vi "Email_With_Log.vi"(0 "recipients":string[](array[string]), 1 "subject ([No Subject])":string="[No Subject]", 2 "message":string, 3 "attachments":T1(array[cluster])) -> (5 "invalid recipients":string[](array[string]), 6 "error out":errorcluster)   [LabVIEW 2010]
uses:
  Globals/Preference_global.vi
  Globals/Constants_global.vi
  <vilib>/Utility/SMTP/NI_SMTPEmail.lvlib
panel:
  out "Number of valid email requests":i32
  # "Image/x-png"
  # "Image/jpeg"
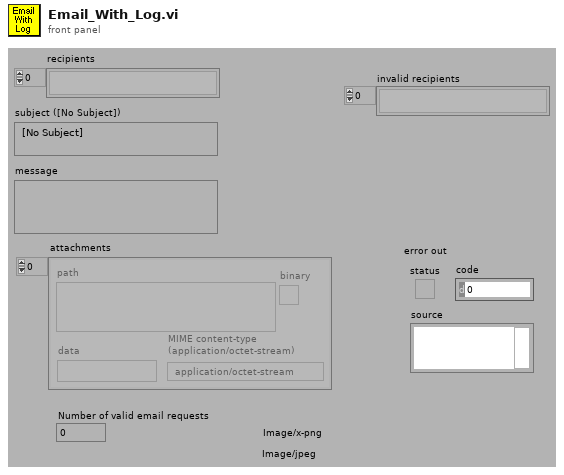
[diagram p1: front panel]
types:
  T1 = cluster{"path":path, "data":string, "binary":bool, "MIME content-type \n(application/octet-stream)":string}[]
  T2 = cluster{"path":path, "data":string, "binary":bool, "MIME content-type \n(application/octet-stream)":string}
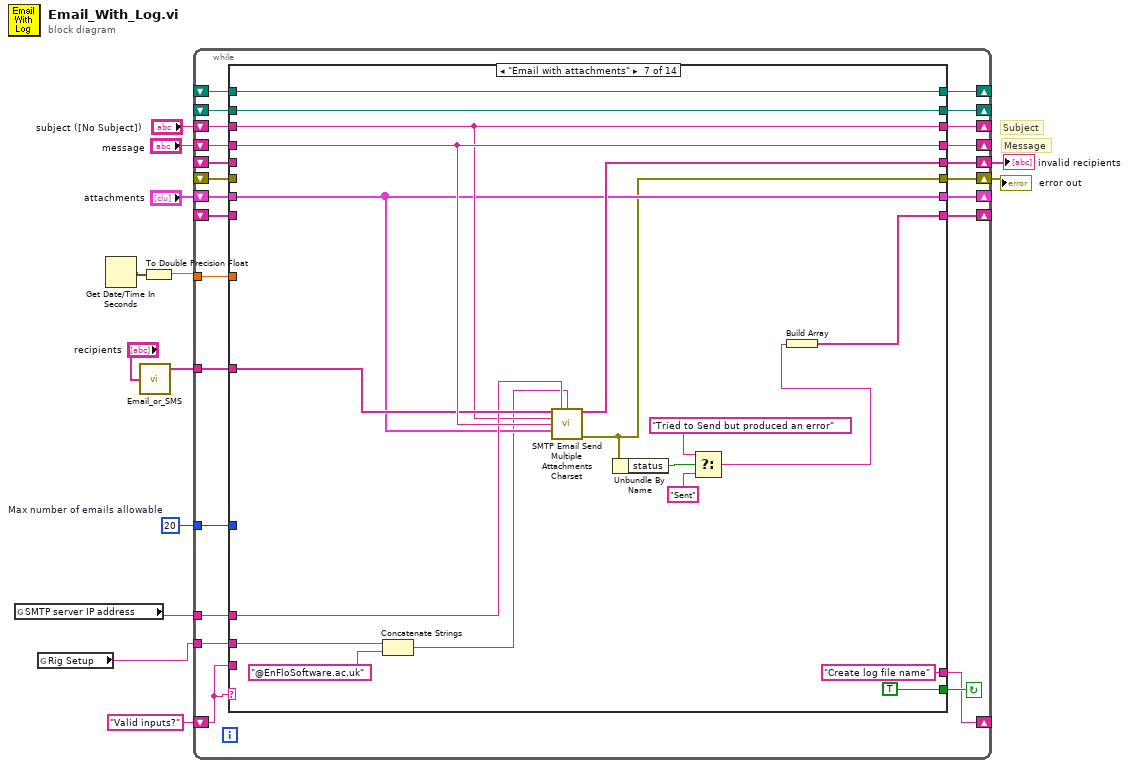
[diagram p0: block diagram]
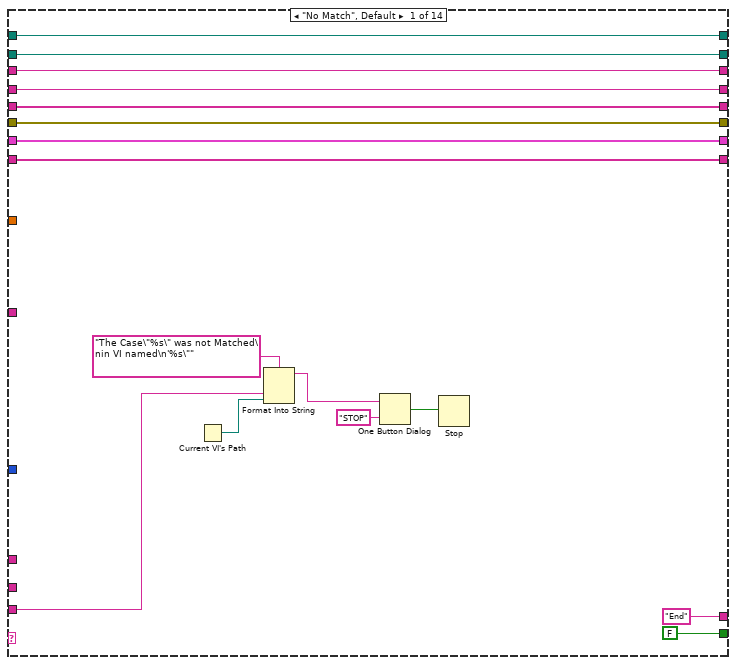
[diagram p2: hidden frame]
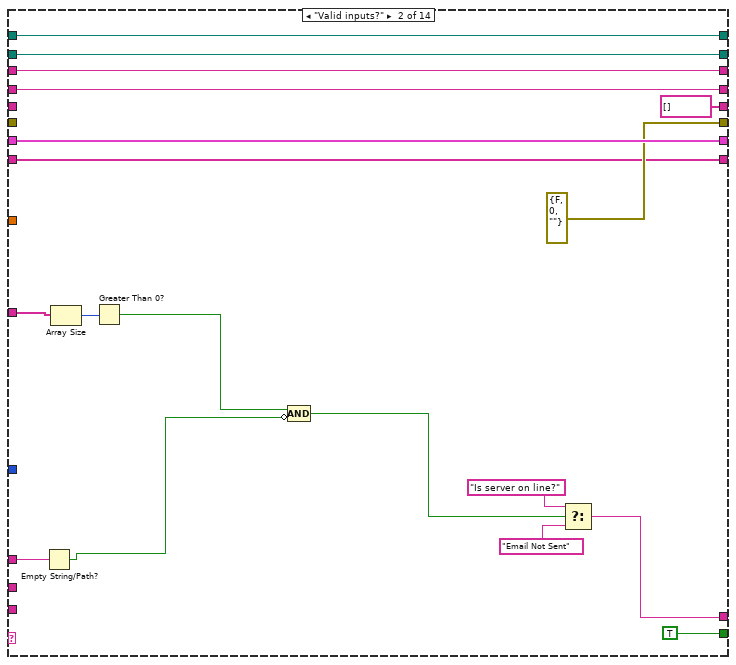
[diagram p3: hidden frame]
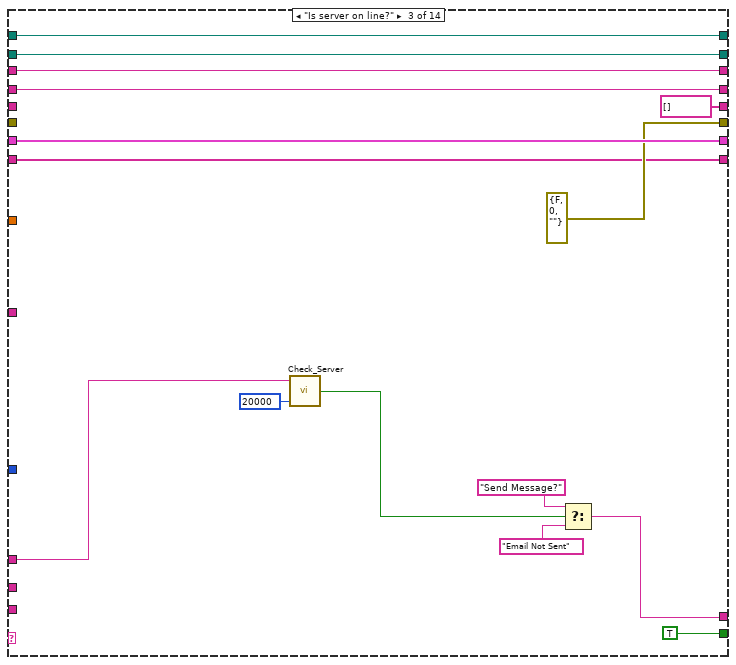
[diagram p4: hidden frame]
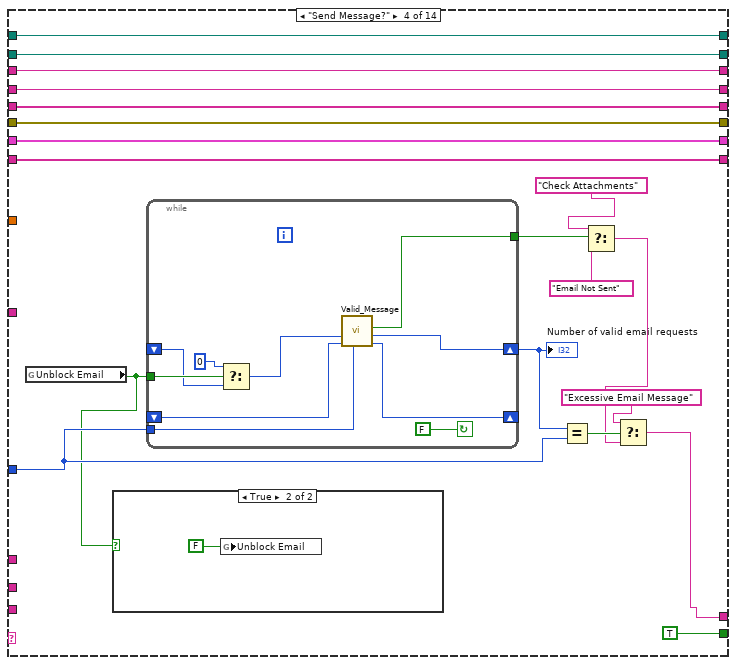
[diagram p5: hidden frame]
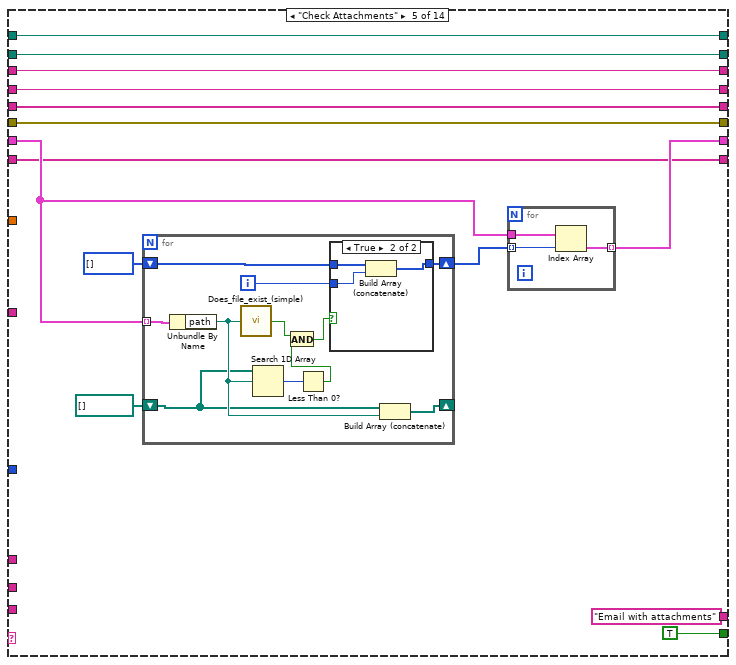
[diagram p7: hidden frame]
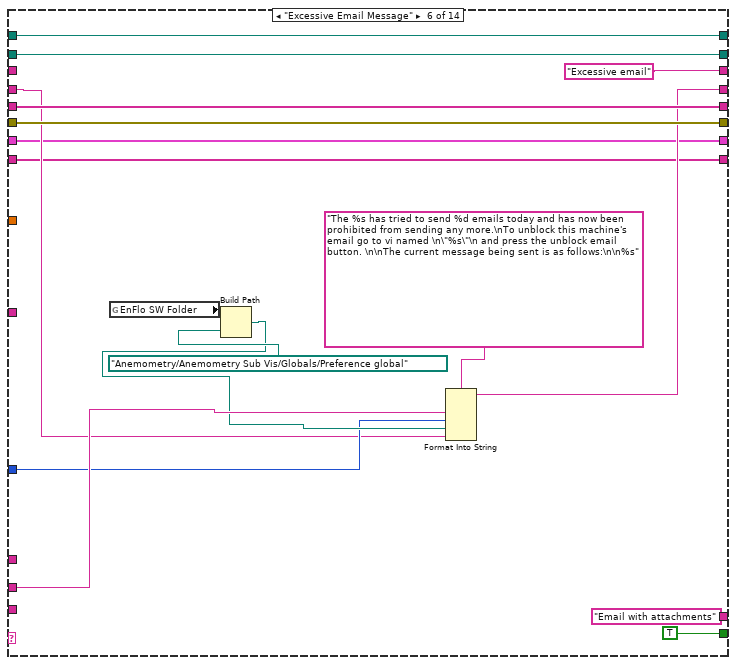
[diagram p9: hidden frame]
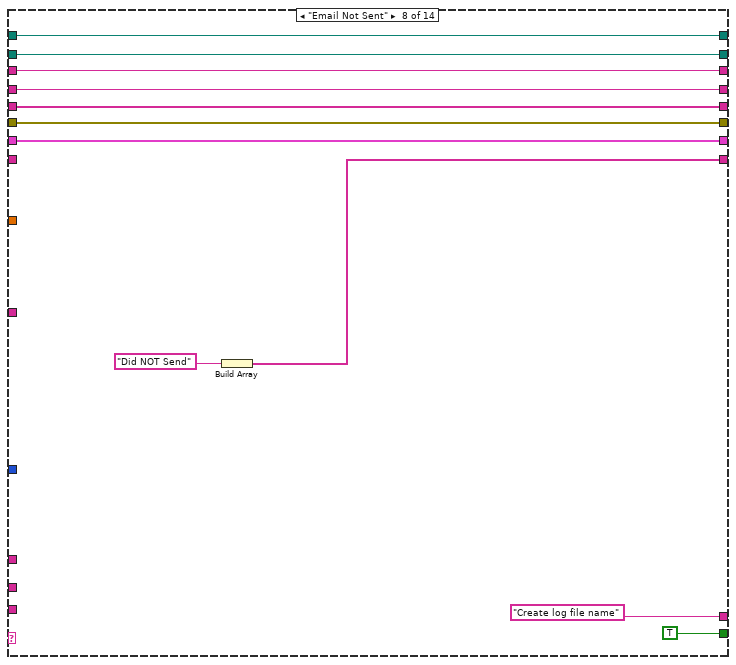
[diagram p10: hidden frame]
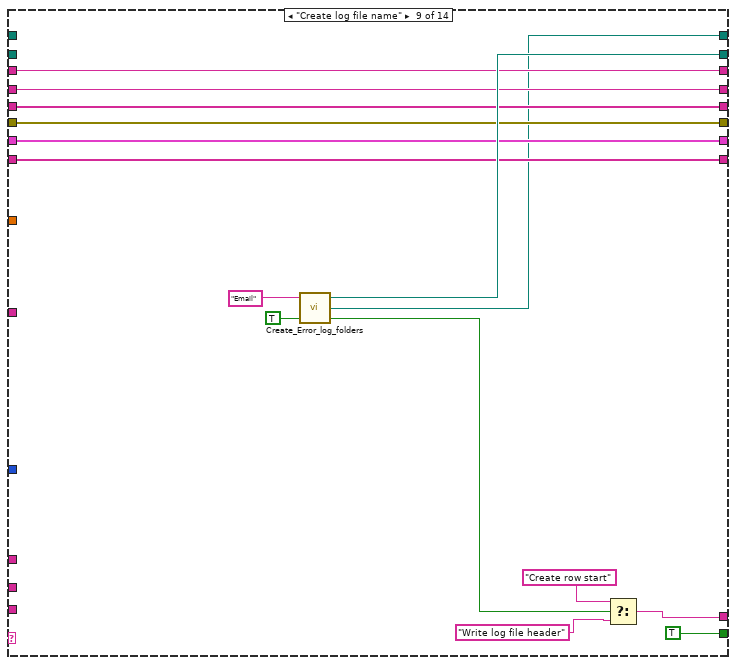
[diagram p11: hidden frame]
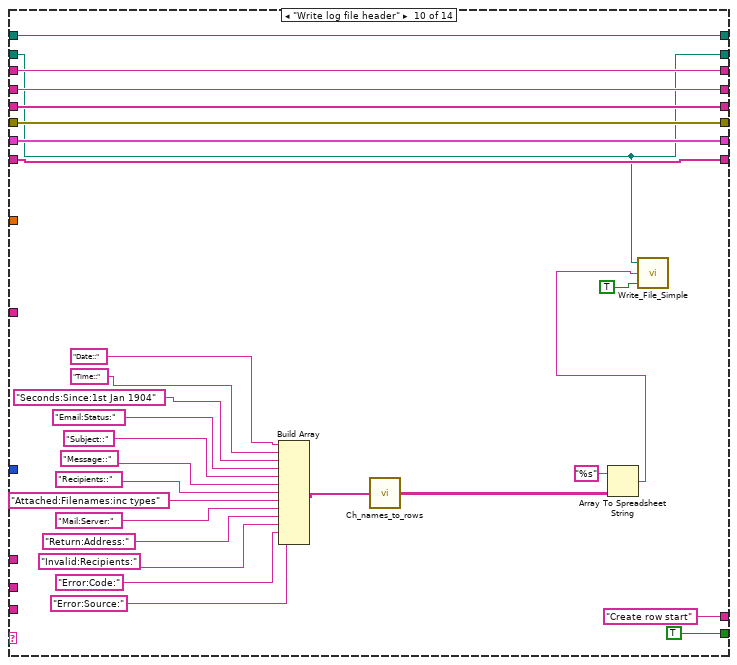
[diagram p12: hidden frame]
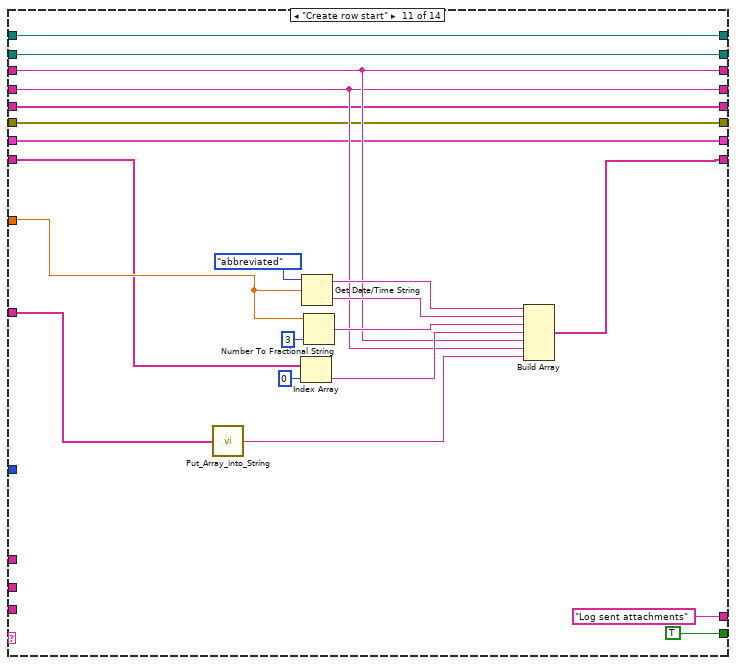
[diagram p13: hidden frame]
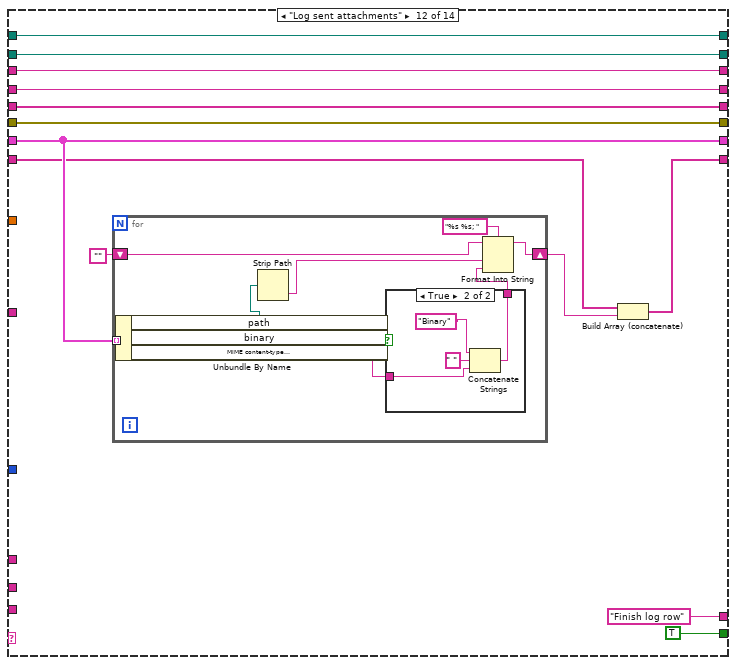
[diagram p14: hidden frame]
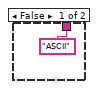
[diagram p15: hidden frame]
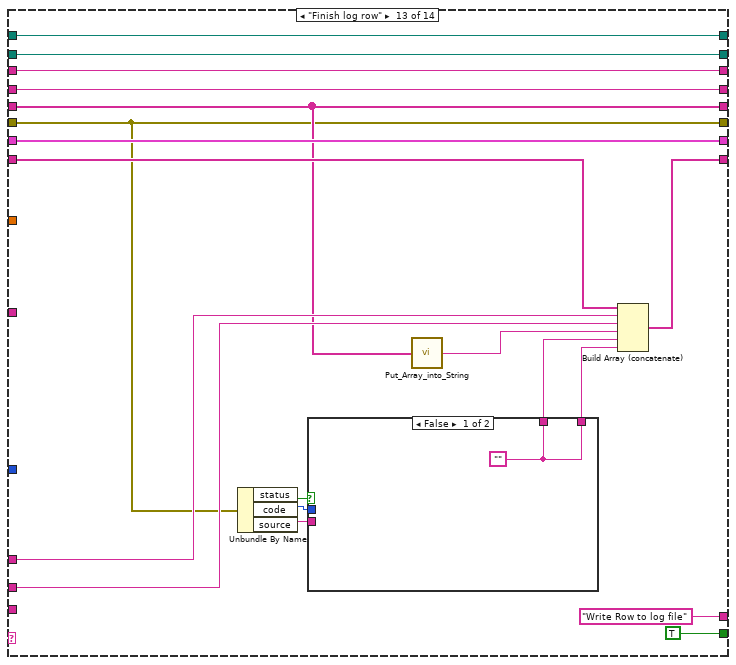
[diagram p16: hidden frame]
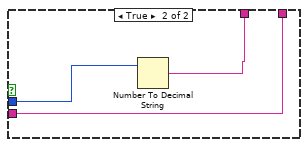
[diagram p17: hidden frame]
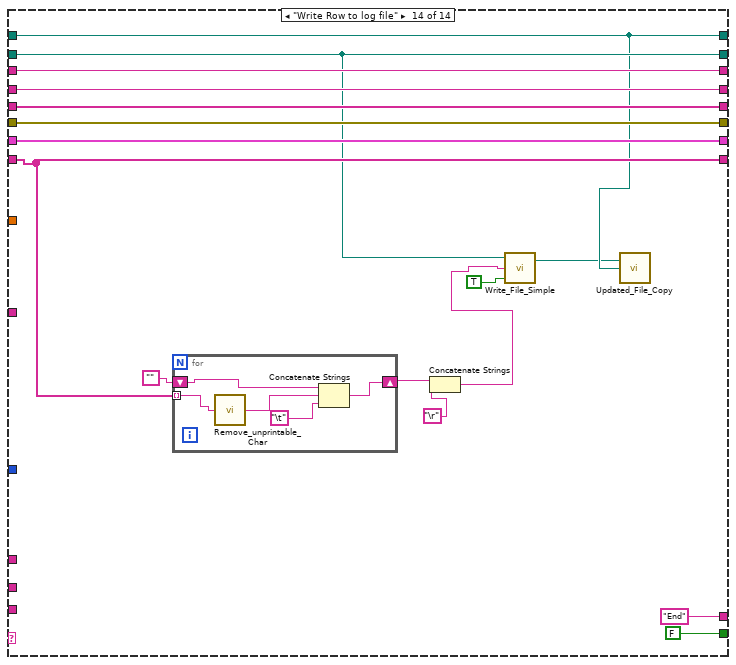
[diagram p18: hidden frame]
diagram:
  w10 = 20  # Max number of emails allowable
  # "Message"
  # "Subject"
  n1 = global read "Preference_global.vi" "SMTP server IP address"() -> (w3:string)
  n2 = global read "Preference_global.vi" "Rig Setup"() -> (w1:string)
  n3 = Get Date/Time In Seconds() -> (seconds since 1Jan1904=w12:timestamp)
  n4 = call "Email_or_SMS.vi"("Email address"="recipients") -> ("Email"=w4:string[])  [unwired: 3 out]
  n5 = To Double Precision Float(number=w12) -> (double precision float=w13:dbl)
  n6 = while {
    tunnel: w13 -> [w35]
    shift-left: "Valid inputs?" -> [w34]
    shift-right: [w36] -> _
    shift-right: [w32] -> _
    shift-left: _ -> [w33]
    tunnel: w10 -> [w31]
    shift-right: [w29] -> _
    shift-left: "subject ([No Subject])" -> [w30]
    shift-right: [w28] -> _
    shift-left: "message" -> [w27]
    shift-right: [w25] -> w8
    shift-left: _ -> [w26]
    shift-right: [w24] -> w2
    shift-left: _ -> [w23]
    tunnel: w1 -> [w22]
    shift-right: [w20] -> _
    shift-left: "attachments" -> [w21]
    tunnel: w4 -> [w19]
    tunnel: w3 -> [w18]
    shift-right: [w17] -> _
    shift-left: _ -> [w16]
    shift-right: [w15] -> _
    shift-left: _ -> [w14]
    stop <- w37 continue-if-true
    n7 = case shown="\"Email with attachments\"" w34 {
      tunnel: [FALSE ("Abort") TRUE ("Abort") TRUE ("Abort") TRUE ("Abort") TRUE ("Abort") TRUE ("Abort") TRUE ("Abort") TRUE ("Abort") TRUE ("status") TRUE TRUE TRUE TRUE FALSE] -> w37
      tunnel: ["End" ("f") w59 w80 w94 "Email with attachments" ("f") "Email with attachments" ("f") "Create log file name" ("f") "Create log file name" ("f") w208 "Create row start" ("f") "Log sent attachments" ("f") "Finish log row" ("f") "Write Row to log file" ("f") "End" ("f")] -> w36
      tunnel: w35 -> [_ _ _ _ _ _ _ _ _ _ w254 _ _ _]
      tunnel: w34 -> [w48 _ _ _ _ _ _ _ _ _ _ _ _ _]
      tunnel: w33 -> [w45 w70 w85 w104 w129 w164 w183 w194 _ w212 w251 w270 w303 w313]
      tunnel: [w45 w70 w85 w104 w129 w164 w183 w194 w205 w212 w251 w270 w303 w313] -> w32
      tunnel: w31 -> [_ _ _ w102 _ w154 _ _ _ _ _ _ _ _]
      tunnel: w30 -> [w44 w69 w84 w101 w128 _ w177 w193 w203 w226 w244 w268 w301 w320]
      tunnel: [w44 w69 w84 w101 w128 "Excessive email" ("Email address") w177 w193 w203 w226 w244 w268 w301 w320] -> w29
      tunnel: [w43 w68 w83 w100 w127 w158 w182 w192 w202 w225 w243 w267 w300 w319] -> w28
      tunnel: w27 -> [w43 w68 w83 w100 w127 w153 w182 w192 w202 w225 w243 w267 w300 w319]
      tunnel: w26 -> [w42 _ _ w99 w126 w163 _ w191 w201 w224 w242 w266 w295 w318]
      tunnel: [w42 string[] [] ("invalid recipients") string[] [] ("invalid recipients") w99 w126 w163 w180 w191 w201 w224 w242 w266 w295 w318] -> w25
      tunnel: [w41 errorcluster {"status"=FALSE, "code"=0, "source"=""} ("error out") errorcluster {"status"=FALSE, "code"=0, "source"=""} ("error out") w98 w125 w162 w175 w190 w200 w223 w241 w265 w293 w317] -> w24
      tunnel: w23 -> [w41 _ _ w98 w125 w162 _ w190 w200 w223 w241 w265 w293 w317]
      tunnel: w22 -> [_ _ _ _ _ w157 w168 _ _ _ _ _ w296 _]
      tunnel: w21 -> [w40 w58 w79 w90 w122 w151 w176 w189 w199 w222 w240 w264 w299 w316]
      tunnel: [w40 w58 w79 w90 w121 w151 w176 w189 w199 w222 w240 w264 w299 w316] -> w20
      tunnel: w19 -> [_ w67 _ _ _ _ w181 _ _ _ w246 _ _ _]
      tunnel: w18 -> [_ w65 w75 _ _ _ w179 _ _ _ _ _ w297 _]
      tunnel: w16 -> [w39 w56 w77 w89 w119 w150 _ _ w198 w215 w250 w261 w298 w315]
      tunnel: [w39 w56 w77 w89 w119 w150 w170 w186 w198 w215 w247 w269 w302 w315] -> w17
      tunnel: [w38 w54 w72 w87 w117 w149 w169 w185 w197 w214 w239 w260 w287 w312] -> w15
      tunnel: w14 -> [w38 w54 w72 w87 w117 w149 w169 w185 _ w214 w239 w260 w287 w312]
      frame "No Match", Default {
        n8 = Current VI's Path() -> (path=w49:path)
        n9 = Format Into String(format string="The Case\"%s\" was not Matched\nin VI named\n'%s\"" ("Format String"), w48, w49) -> (resulting string=w52:string)  [unwired: 2 in, 1 out]
        n10 = One Button Dialog(message=w52, button name ("OK")="STOP") -> (true=w50:bool)
        n11 = Stop(stop? (T)=w50) -> ()
      }
      frame "Valid inputs?" {
        n12 = Empty String/Path?(string/path=w65) -> (empty?=w63:bool)
        n13 = Array Size(array=w67) -> (size(s)=w66:i32)
        n14 = Greater Than 0?(x=w66) -> (x > 0?=w64:bool)
        n15 = Compound Arithmetic op=AND(w64, invert w63) -> (w62:bool)
        n16 = Select(t="Is server on line?" ("f"), s=w62, f="Email Not Sent") -> (s? t:f=w59:string)
      }
      frame "Is server on line?" {
        n17 = call "Check_Server.vi"("timeout ms (60000)"=20000, "address"=w75) -> ("OK"=w74:bool)  [unwired: 3 out]
        n18 = Select(t="Send Message?" ("f"), s=w74, f="Email Not Sent") -> (s? t:f=w80:string)
      }
      frame "Send Message?" {
        n19 = global read "Preference_global.vi" "Unblock Email"() -> (w88:bool)
        n20 = case shown="True" w88 {
          frame False {
          }
          frame True {
            n21 = global write "Preference_global.vi" "Unblock Email"(FALSE ("Unblock Email")) -> ()
          }
        }
        n22 = while {
          tunnel: w88 -> [w111]
          tunnel: w102 -> [w113]
          tunnel: [w114] -> w96
          shift-left: _ -> [w110]
          shift-right: [w112] -> w103
          shift-left: _ -> [w116]
          shift-right: [w115] -> _
          stop <- FALSE continue-if-true
          n23 = Select(t=0, s=w111, f=w110) -> (s? t:f=w109:i32)
          n24 = call "Valid_Message.vi"("Max per day"=w113, "day of month in"=w116, "Number of requests today In"=w109) -> ("day of month out"=w115:i32, "Number of requests today Out"=w112:i32, "Send Message"=w114:bool)  [unwired: 2 in, 4 out]
        }
        "Number of valid email requests" <- w103
        n25 = Equal?(x=w103, y=w102) -> (x = y?=w97:bool)
        n26 = Select(t="Check Attachments", s=w96, f="Email Not Sent") -> (s? t:f=w95:string)
        n27 = Select(t="Excessive Email Message", s=w97, f=w95) -> (s? t:f=w94:string)
      }
      frame "Check Attachments" {
        n28 = for {
          tunnel: w122 -> [w144] mode=indexing
          shift-right: [w141] -> w123
          shift-left: i32[] [] -> [w143]
          shift-right: [w140] -> _
          shift-left: path[] [] -> [w138]
          i -> [w142]
          n29 = Unbundle By Name(w144) -> ("path"=w139:path)
          n30 = call "Does_file_exist_(simple).vi"("Pathname"=w139) -> ("exists?"=w136:bool)
          n31 = Search 1D Array(1D array=w138, element=w139) -> (index of element=w137:i32)  [unwired: 1 out]
          n32 = Less Than 0?(x=w137) -> (x < 0?=w135:bool)
          n33 = And(x=w136, y=w135) -> (x .and. y?=w134:bool)
          n34 = case shown="True" w134 {
            tunnel: w143 -> [w145 w148]
            tunnel: w142 -> [_ w147]
            tunnel: [w145 w146] -> w141
            frame False {
            }
            frame True {
              n35 = Build Array (concatenate)(w148, w147) -> (w146:i32[])
            }
          }
          n36 = Build Array (concatenate)(w138, w139) -> (w140:path[])
        }
        n37 = for {
          tunnel: w123 -> [w133] mode=indexing
          tunnel: w122 -> [w132]
          tunnel: [w131] -> w121 mode=indexing
          n38 = Index Array(array=w132, index=w133) -> (element=w131:T2)
        }
      }
      frame "Excessive Email Message" {
        n39 = global read "Constants_global.vi" "EnFlo SW Folder"() -> (w160:path)
        n40 = Build Path(base path=w160, name or relative path=path "Anemometry/Anemometry Sub Vis/Globals/Preference global") -> (appended path=w156:path)
        n41 = Format Into String(format string="The %s has tried to send %d emails today and has now been prohibited from sending any more.\nTo unblock this machine's email go to vi named \n\"%s\"\n and press the unblock email button. \n\nThe current message being sent is as follows:\n\n%s" ("Format String"), w157, w154, w156, w153) -> (resulting string=w158:string)  [unwired: 2 in, 1 out]
      }
      frame "Email with attachments" {
        n42 = Concatenate Strings(w168, "@EnFloSoftware.ac.uk" ("string")) -> (w167:string)
        n43 = call <vilib>:"SMTP Email Send Multiple Attachments Charset.vi"("recipients"=w181, "mail server"=w179, "return address"=w167, "subject ([No Subject])"=w177, "message"=w182, "attachments"=w176) -> ("invalid recipients"=w180:string[], "error out"=w175:errorcluster)  [unwired: 2 in, 6 out]
        n44 = Unbundle By Name(w175) -> ("status"=w174:bool)
        n45 = Select(t="Tried to Send but produced an error", s=w174, f="Sent") -> (s? t:f=w171:string)
        n46 = Build Array(w171) -> (w170:string[])
      }
      frame "Email Not Sent" {
        n47 = Build Array("Did NOT Send") -> (w186:string[])
      }
      frame "Create log file name" {
        n48 = call "Create_Error_log_folders.vi"("Per Day Log File?"=TRUE, "Log Filename"="Email" ("Input Element")) -> ("exists?"=w204:bool, "Server copy Location"=w197:path, "Local Log File"=w205:path)  [unwired: 1 in]
        n49 = Select(t="Create row start", s=w204, f="Write log file header") -> (s? t:f=w208:string)
      }
      frame "Write log file header" {
        n50 = Build Array("Date::", "Time::", "Seconds:Since:1st Jan 1904", "Email:Status:", "Subject::", "Message::", "Recipients::", "Attached:Filenames:inc types", "Mail:Server:", "Return:Address:", "Invalid:Recipients:", "Error:Code:", "Error:Source:") -> (w233:string[])
        n51 = call "Ch_names_to_rows.vi"("Channel Names"=w233) -> ("3 Row names"=w232:string[][])
        n52 = Array To Spreadsheet String(array=w232, 3:"%s" ("format string")) -> (spreadsheet string=w211:string)  [unwired: 1 out]
        n53 = call "Write_File_Simple.vi"("append to file? (new file:F)"=TRUE, "character string"=w211, "file path"=w212) -> ()  [unwired: 2 out]
      }
      frame "Create row start" {
        n54 = call "Put_Array_into_String.vi"("String array"=w246) -> ("String Value"=w245:string)
        n55 = Index Array(array=w250, index=0) -> (element=w248:string)
        n56 = Get Date/Time String(date format (0)=enum16{"short", "long", "abbreviated"}."abbreviated", seconds (now)=w254) -> (date string=w258:string, time string=w257:string)  [unwired: 1 out]
        n57 = Number To Fractional String(number=w254, precision (6)=i16 3) -> (F-format string=w253:string)  [unwired: 2 out]
        n58 = Build Array(w258, w257, w253, w248, w244, w243, w245) -> (w247:string[])
      }
      frame "Log sent attachments" {
        n59 = for {
          tunnel: w264 -> [w281] mode=indexing
          shift-right: [w275] -> w262
          shift-left: "" -> [w276]
          n60 = Unbundle By Name(w281) -> ("path"=w280:path, "binary"=w278:bool, "MIME content-type \n(application/octet-stream)"=w277:string)
          n61 = Strip Path(path=w280) -> (name=w279:string)  [unwired: 1 out]
          n62 = case shown="True" w278 {
            tunnel: w277 -> [_ w284]
            tunnel: ["ASCII" w283] -> w274
            frame False {
            }
            frame True {
              n63 = Concatenate Strings("Binary", " " ("string"), w284) -> (w283:string)
            }
          }
          n64 = Format Into String(format string="%s %s; ", initial string=w276, w279, w274) -> (resulting string=w275:string)  [unwired: 1 in, 1 out]
        }
        n65 = Build Array (concatenate)(w261, w262) -> (w269:string[])
      }
      frame "Finish log row" {
        n66 = Unbundle By Name(w293) -> ("status"=w292:bool, "code"=w291:i32, "source"=w290:string)
        n67 = case shown="False" w292 {
          tunnel: w291 -> [_ w308]
          tunnel: w290 -> [_ w309]
          tunnel: [w306 w309] -> w289
          tunnel: [w306 w307] -> w288
          frame False {
            w306 = ""
          }
          frame True {
            n68 = Number To Decimal String(number=w308) -> (decimal integer string=w307:string)  [unwired: 1 out]
          }
        }
        n69 = call "Put_Array_into_String.vi"("String array"=w295) -> ("String Value"=w294:string)
        n70 = Build Array (concatenate)(w298, w297, w296, w294, w288, w289) -> (w302:string[])
      }
      frame "Write Row to log file" {
        n71 = for {
          shift-right: [w329] -> w321
          shift-left: "" -> [w330]
          tunnel: w315 -> [w327] mode=indexing
          n72 = call "Remove_unprintable_Char.vi"("Input String"=w327) -> ("Output String"=w326:string)
          n73 = Concatenate Strings(w330, w326, "\t") -> (w329:string)
        }
        n74 = Concatenate Strings(w321, "\r") -> (w314:string)
        n75 = call "Write_File_Simple.vi"("append to file? (new file:F)"=TRUE, "character string"=w314, "file path"=w313) -> ("file path Out"=w310:path)  [unwired: 1 out]
        n76 = call "Updated_File_Copy.vi"("Target Path"=w312, "Source Path"=w310) -> ()  [unwired: 2 out]
      }
    }
  }
  "invalid recipients" <- w8
  "error out" <- w2
